vi "data_input.vi"() -> (4 "\"y\" value output":dbl, 10 "Done output":bool, 15 "Finish output":bool)   [LabVIEW 2018]
panel:
  in  "Done":bool
  in  "Finish":bool
  in  "y_value":string caption="\"y\" value"
  # "el scan fov 0 y"
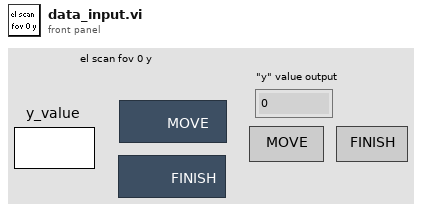
[diagram p1: front panel]
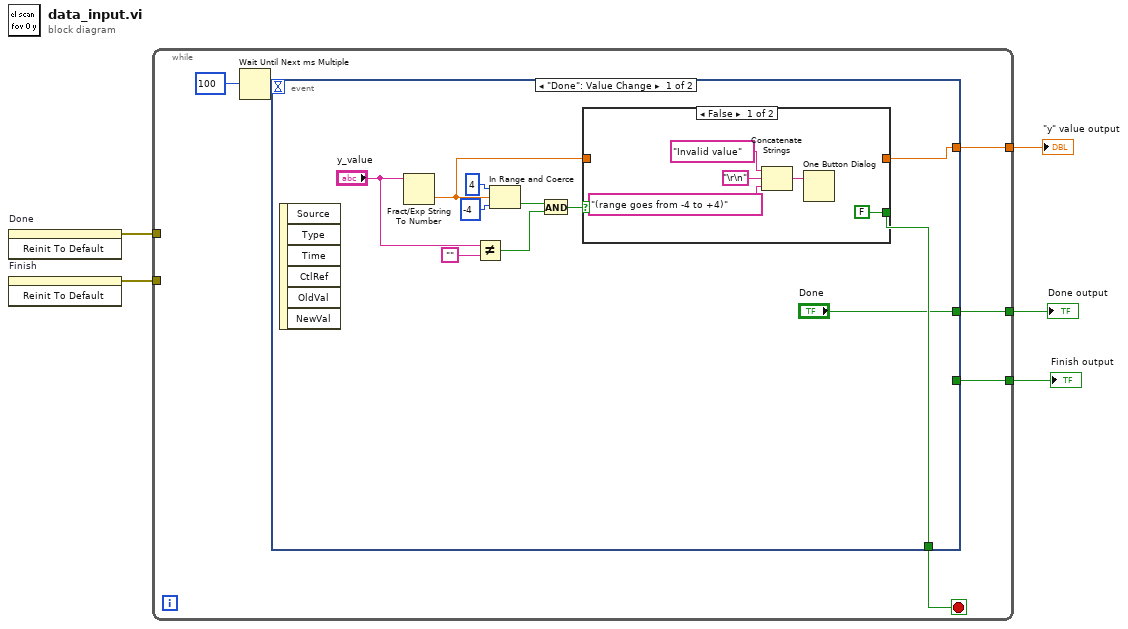
[diagram p0: block diagram]
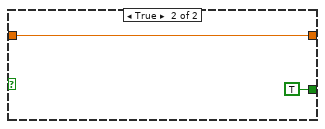
[diagram p2: hidden frame]
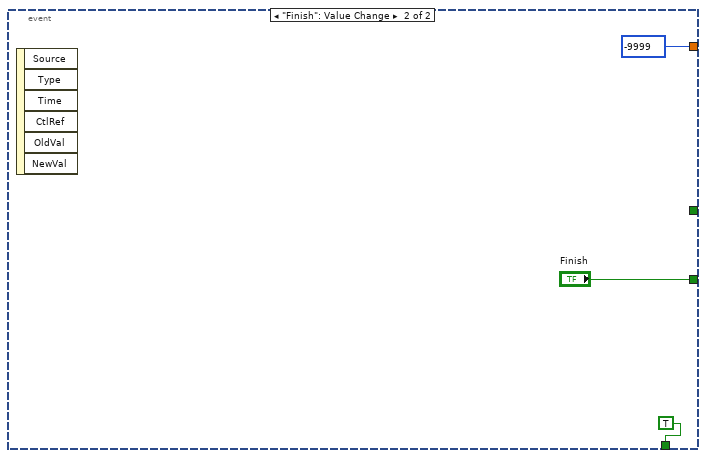
[diagram p3: hidden frame]
diagram:
  n1 = invoke on="Done" class="Bool" method="Reinit To Default"() -> (error out=w4:errorcluster)  [unwired: 3 in, 2 out]
  n2 = invoke on="Finish" class="Bool" method="Reinit To Default"() -> (error out=w5:errorcluster)  [unwired: 3 in, 2 out]
  n3 = while {
    tunnel: [w10] -> w3
    tunnel: w4 -> [_]
    tunnel: w5 -> [_]
    tunnel: [w7] -> w2
    tunnel: [w6] -> w1
    stop <- w8 stop-if-true
    n4 = Wait Until Next ms Multiple(millisecond multiple=100) -> ()  [unwired: 1 out]
    n5 = event shown="[0] \"Done\": Value Change" {
      selector: _ -> [_ _]
      dyn-events: _ -> [_ _]
      timeout: _ -> [_ _]
      tunnel: [w18 TRUE] -> w8
      tunnel: [w19 -9999 ("upper limit")] -> w10
      tunnel: ["Done" _] -> w7
      tunnel: [_ "Finish"] -> w6
      event "Done": Value Change {
        n6 = event-data() -> ()  [unwired: 7 out]
        n7 = Fract/Exp String To Number(string="y_value") -> (number=w17:dbl)  [unwired: 3 in, 1 out]
        n8 = Not Equal?(x="y_value", y="") -> (x != y?=w11:bool)
        n9 = In Range and Coerce(upper limit=4, x=w17, lower limit=-4) -> (In Range?=w13:bool)  [unwired: 1 out]
        n10 = And(x=w13, y=w11) -> (x .and. y?=w12:bool)
        n11 = case shown="False" w12 {
          tunnel: [_ w28] -> w19
          tunnel: w17 -> [_ w28]
          tunnel: [FALSE TRUE] -> w18
          frame False {
            n12 = Concatenate Strings("Invalid value" ("message"), "\r\n", "(range goes from -4 to +4)" ("message")) -> (w23:string)
            n13 = One Button Dialog(message=w23) -> ()  [unwired: 1 in, 1 out]
          }
          frame True {
          }
        }
      }
      event "Finish": Value Change {
        n14 = event-data() -> ()  [unwired: 7 out]
      }
    }
  }
  "\"y\" value output" <- w3
  "Done output" <- w2
  "Finish output" <- w1
